vi "X1000.vi"(1 "X":dbl) -> (0 "X/1000":dbl)   [LabVIEW 2020]
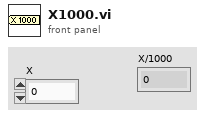
[diagram p1: front panel]
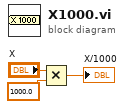
[diagram p0: block diagram]
diagram:
  n1 = Multiply(x="X", y=1000.0) -> (x*y=→"X/1000":dbl)
